vi "Clear.vi"(8 "error in (no error)":errorcluster, 11 "64x128 I2C OLED SSD1315 In":refnum<class "64x128 I2C OLED SSD1315.lvclass">) -> (0 "error out":errorcluster, 2 "2D Picture":picture, 3 "64x128 I2C OLED SSD1315 Out":refnum<class "64x128 I2C OLED SSD1315.lvclass">)   [LabVIEW 2020, in "CTI-Peripheral.lvlib" / "64x128 I2C OLED SSD1315.lvclass"]
uses:
  64x128 I2C OLED SSD1315.lvclass
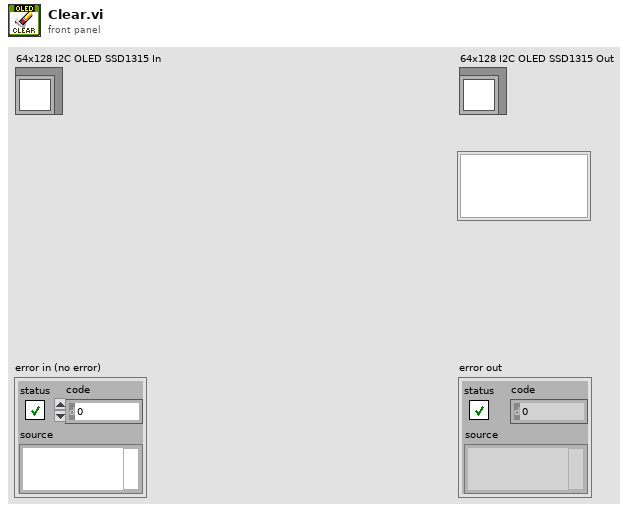
[diagram p1: front panel]
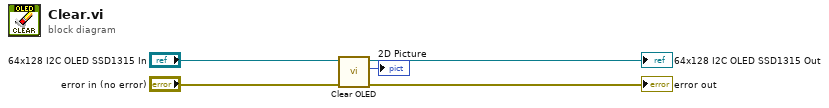
[diagram p0: block diagram]
diagram:
  n1 = call "Clear OLED.vi"("error in (no error)"="error in (no error)", "64x128 I2C OLED SSD1315 in"="64x128 I2C OLED SSD1315 In") -> ("error out"=→"error out":errorcluster, "2D Picture"=→"2D Picture":picture, "64x128 I2C OLED SSD1315 out"=→"64x128 I2C OLED SSD1315 Out":refnum<class "64x128 I2C OLED SSD1315.lvclass">)  [unwired: 7 in]
